vi "Initialize Attributes.vi"(8 "Error In":errorcluster, 10 "Attribute Data":variant, 11 "TestLNA in":refnum<class "TestLNA.lvclass">) -> (0 "Error Out":errorcluster, 2 "Found?":bool, 3 "TestLNA out":refnum<class "TestLNA.lvclass">)   [LabVIEW 2014, in "TestLNA.lvlib" / "TestLNA.lvclass"]
doc: "Initialize object attribute.\n\nUnique resources should be allocated elsewhere!"
uses:
  TestLNA.lvclass
  TestLNA.lvclass/TestLNA.ctl
  CSPP_Core/Actors/CS++BaseActor/CS++BaseActor.lvclass
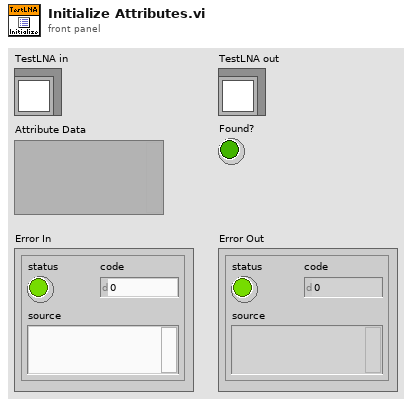
[diagram p1: front panel]
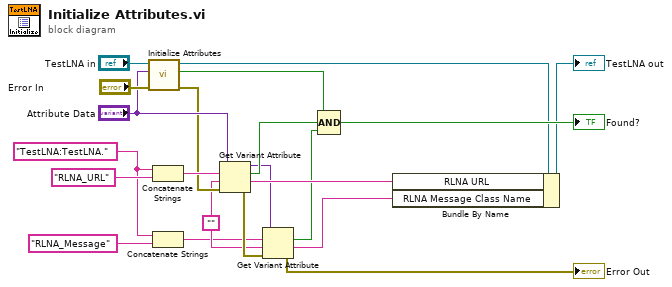
[diagram p0: block diagram]
diagram:
  w7 = ""
  w5 = "TestLNA:TestLNA."
  n1 = call-parent "Initialize Attributes.vi"("error in (no error)"="Error In", "Attribute Data"="Attribute Data", "CS++BaseActor in"="TestLNA in") -> ("error out"=w12:errorcluster, "Found?"=w21:bool, "CS++BaseActor out"=w11:refnum<class "TestLNA.lvclass">)  [unwired: 6 in]
  n2 = Concatenate Strings(w5, "RLNA_URL" ("string")) -> (w16:string)
  n3 = Concatenate Strings(w5, "RLNA_Message" ("string")) -> (w4:string)
  n4 = Get Variant Attribute(Variant="Attribute Data", name=w16, default value (empty Variant)=w7, error in=w12) -> (duplicate Variant=w9:variant, found=w13:bool, value=w15:string, error out=w8:errorcluster)
  n5 = Get Variant Attribute(Variant=w9, name=w4, default value (empty Variant)=w7, error in=w8) -> (found=w3:bool, value=w2:string, error out=→"Error Out":errorcluster)  [unwired: 1 out]
  n6 = Compound Arithmetic op=AND(w21, w13, w3) -> (→"Found?":bool)
  n7 = Bundle By Name(cluster=w11, "RLNA URL"=w15, "RLNA Message Class Name"=w2) -> (→"TestLNA out":refnum<class "TestLNA.lvclass">)
